vi "SW_Load_data_for_Analysis.vi"(0 "Data flow controls":T4, 1 "Cluster of paths input":T3, 4 "Progress bar reference":refnum<vi>, 5 "error in (no error)":errorcluster) -> (6 "Data column names":string[](array[string]), 7 "Stimulus presets array (loaded)":T2(array[cluster]), 8 "TTL inputs":u8[](array[numeric]), 9 "TTL outputs":u8[](array[numeric]), 10 "Absolute timestamp":dbl[](array[numeric]), 11 "Zones preference array (loaded)":dbl[][](array[numeric]), 12 "Relative timestamp":dbl[](array[numeric]), 14 "X coord":dbl[](array[numeric]), 15 "Y coord":dbl[](array[numeric]), 16 "Loaded data":T1={"Zones preference array (loaded)"=[], "TTL inputs"=[], "TTL outputs"=[], "Stimulus presets array (loaded)"=[], "Absolute timestamp"=[], "Relative timestamp"=[], "X coord"=[], "Y coord"=[], "alpha rot. angle"=[], "Current zone"=[], "Acquisition settings cluster out"={"Researcher name"="", "N segments MIDFIELD"=0, "N segments BORDER"=0, "Radius, mm CENTER"=0, "Radius, mm MIDFIELD"=0, "Starting angle MIDFIELD"=0, "Starting angle BORDER"=0, "Cage diameter, mm"=0, "Bridge swap"=FALSE, "Bridge V. offset"=0.0, "Twisted neck"=FALSE, "Offset H."=0.0, "Name prefix"="SavedTrack", "Stop at"=0.0, "\"Stop at\" enabled"=FALSE, "Settings loaded OK"=FALSE}, "Data column names"=[]} {"Acquisition settings cluster out"."Stop at" format="%<%H:%M:%S>t"}, 17 "alpha rot. angle":dbl[](array[numeric]), 18 "Current zone":dbl[](array[numeric]), 19 "error out":errorcluster)   [LabVIEW 2018, in "Tracker.lvlib"]
uses:
  <extravilib>/ChannelInstances/Stream-a[.,.](dbl)/Read With Abort.vi
  <extravilib>/ChannelInstances/Stream-a[.,.](dbl)/Write With Abort.vi
  <extravilib>/ChannelInstances/Stream-a[.,.](dbl)/EndpointRead.vi
  <extravilib>/ChannelInstances/Stream-a[.,.](dbl)/Endpoint.vi
  <vilib>/Utility/file.llb/Read Delimited Spreadsheet (string).vi
  <extravilib>/ChannelInstances/Stream-a[.,.](dbl)/Instantiate.vi
  <extravilib>/ChannelInstances/Stream-a[.,.](dbl)/)Channel.vi
  <resource>/ChannelSupport/_ChannelSupport/WaitIfNeeded.vi
  Tracker.lvlib
  <vilib>/Utility/config.llb/NI_LVConfig.lvlib
  <extravilib>/ChannelInstances/Stream-a[.,.](dbl).lvlib
panel:
  out "Settings loaded OK":bool
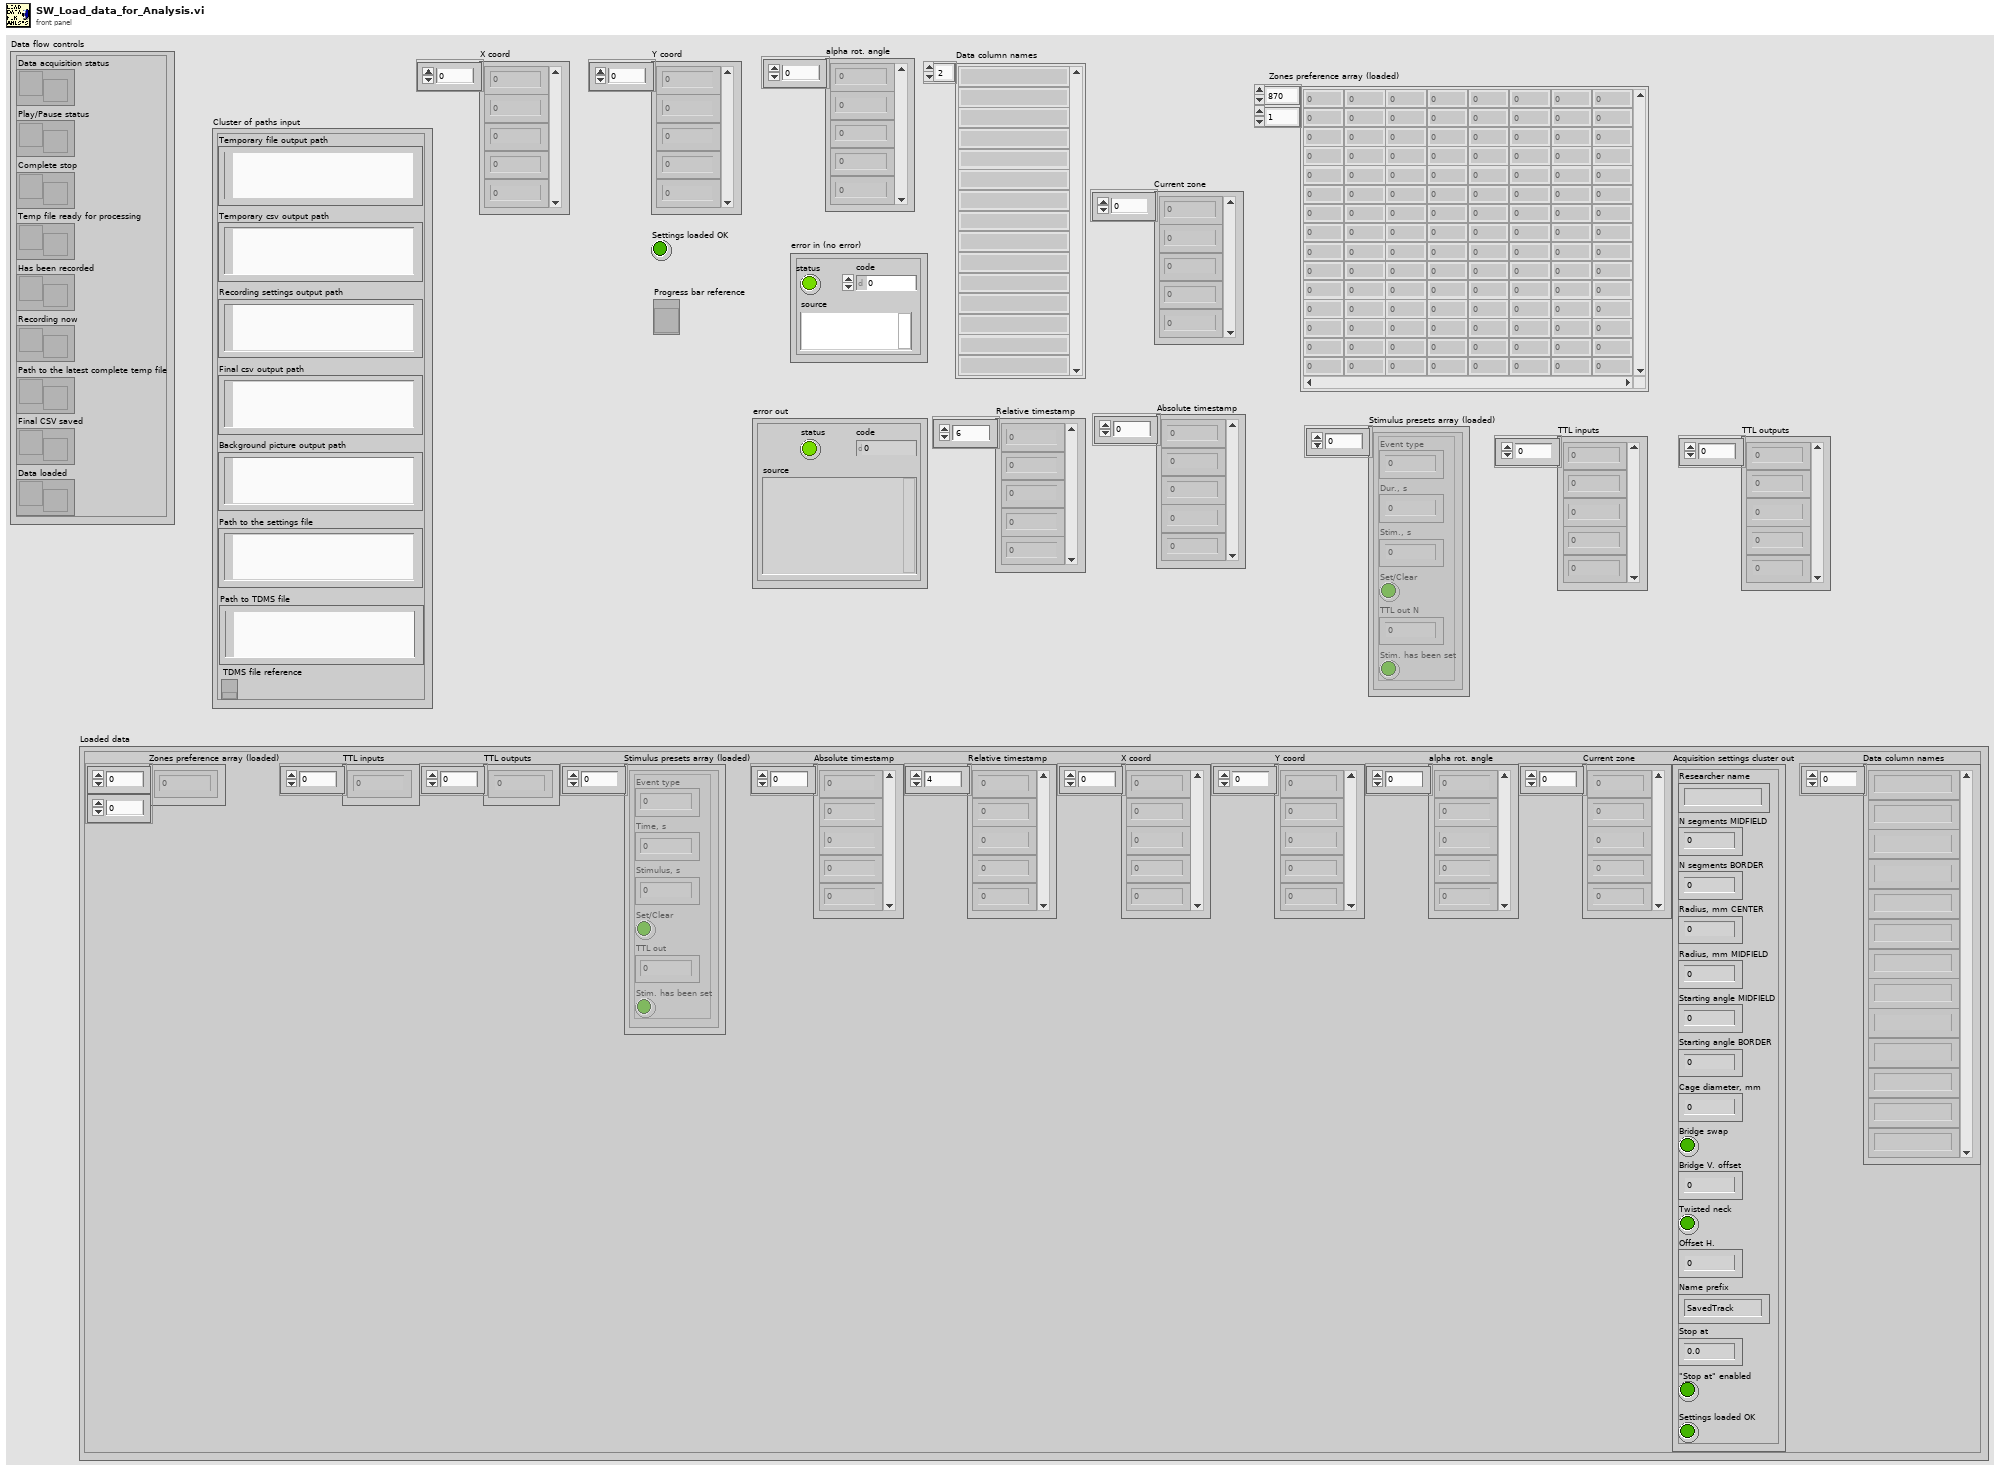
[diagram p1: front panel]
types:
  T1 = cluster{"Zones preference array (loaded)":dbl[][], "TTL inputs":u8[], "TTL outputs":u8[], "Stimulus presets array (loaded)":cluster{"Event type":u16, "Time, s":sgl, "Stimulus, s":sgl, "Set/Clear":bool, "TTL out":u16, "Stim. has been set":bool}[], "Absolute timestamp":dbl[], "Relative timestamp":dbl[], "X coord":dbl[], "Y coord":dbl[], "alpha rot. angle":dbl[], "Current zone":dbl[], "Acquisition settings cluster out":cluster{"Researcher name":string, "N segments MIDFIELD":u8, "N segments BORDER":u8, "Radius, mm CENTER":u16, "Radius, mm MIDFIELD":u16, "Starting angle MIDFIELD":i16, "Starting angle BORDER":i16, "Cage diameter, mm":u16, "Bridge swap":bool, "Bridge V. offset":sgl, "Twisted neck":bool, "Offset H.":sgl, "Name prefix":string, "Stop at":dbl, "\"Stop at\" enabled":bool, "Settings loaded OK":bool}, "Data column names":string[]}
  T2 = cluster{"Event type":u16, "Dur., s":sgl, "Stim., s":sgl, "Set/Clear":bool, "TTL out N":u16, "Stim. has been set":bool}[]
  T3 = cluster{"Temporary file output path":path, "Temporary csv output path":path, "Recording settings output path":path, "Final csv output path":path, "Background picture output path":path, "Path to the settings file":path, "Path to TDMS file":path, "TDMS file reference":refnum<k34>}
  T4 = cluster{"Data acquisition status":refnum<notifier>, "Play/Pause status":refnum<notifier>, "Complete stop":refnum<notifier>, "Temp file ready for processing":refnum<notifier>, "Has been recorded":refnum<notifier>, "Recording now":refnum<notifier>, "Path to the latest complete temp file":refnum<notifier>, "Final CSV saved":refnum<notifier>, "Data loaded":refnum<notifier>}
  T5 = typedef "NI_LVConfig.lvlib/Config Data RefNum.ctl" = refnum<k1>
  T6 = typedef "Stream-a[.,.](dbl).lvlib/)Channel.ctl" = refnum<queue>
  T7 = cluster{"Event type":u16, "Time, s":sgl, "Stimulus, s":sgl, "Set/Clear":bool, "TTL out":u16, "Stim. has been set":bool}
  T8 = cluster{"value":string, "value":u32, "value":u32, "value":u32, "value":u32, "value":i32, "value":i32, "value":u32, "value":bool, "value":dbl, bool, dbl, "key":string, dbl, bool, bool}
  T9 = cluster{"element":dbl[][], u8[], u8[], cluster{"Event type":u16, "Time, s":sgl, "Stimulus, s":sgl, "Set/Clear":bool, "TTL out":u16, "Stim. has been set":bool}[], dbl[], dbl[], dbl[], dbl[], dbl[], dbl[], cluster{"value":string, "value":u32, "value":u32, "value":u32, "value":u32, "value":i32, "value":i32, "value":u32, "value":bool, "value":dbl, bool, dbl, "key":string, dbl, bool, bool}, "first row":string[]}
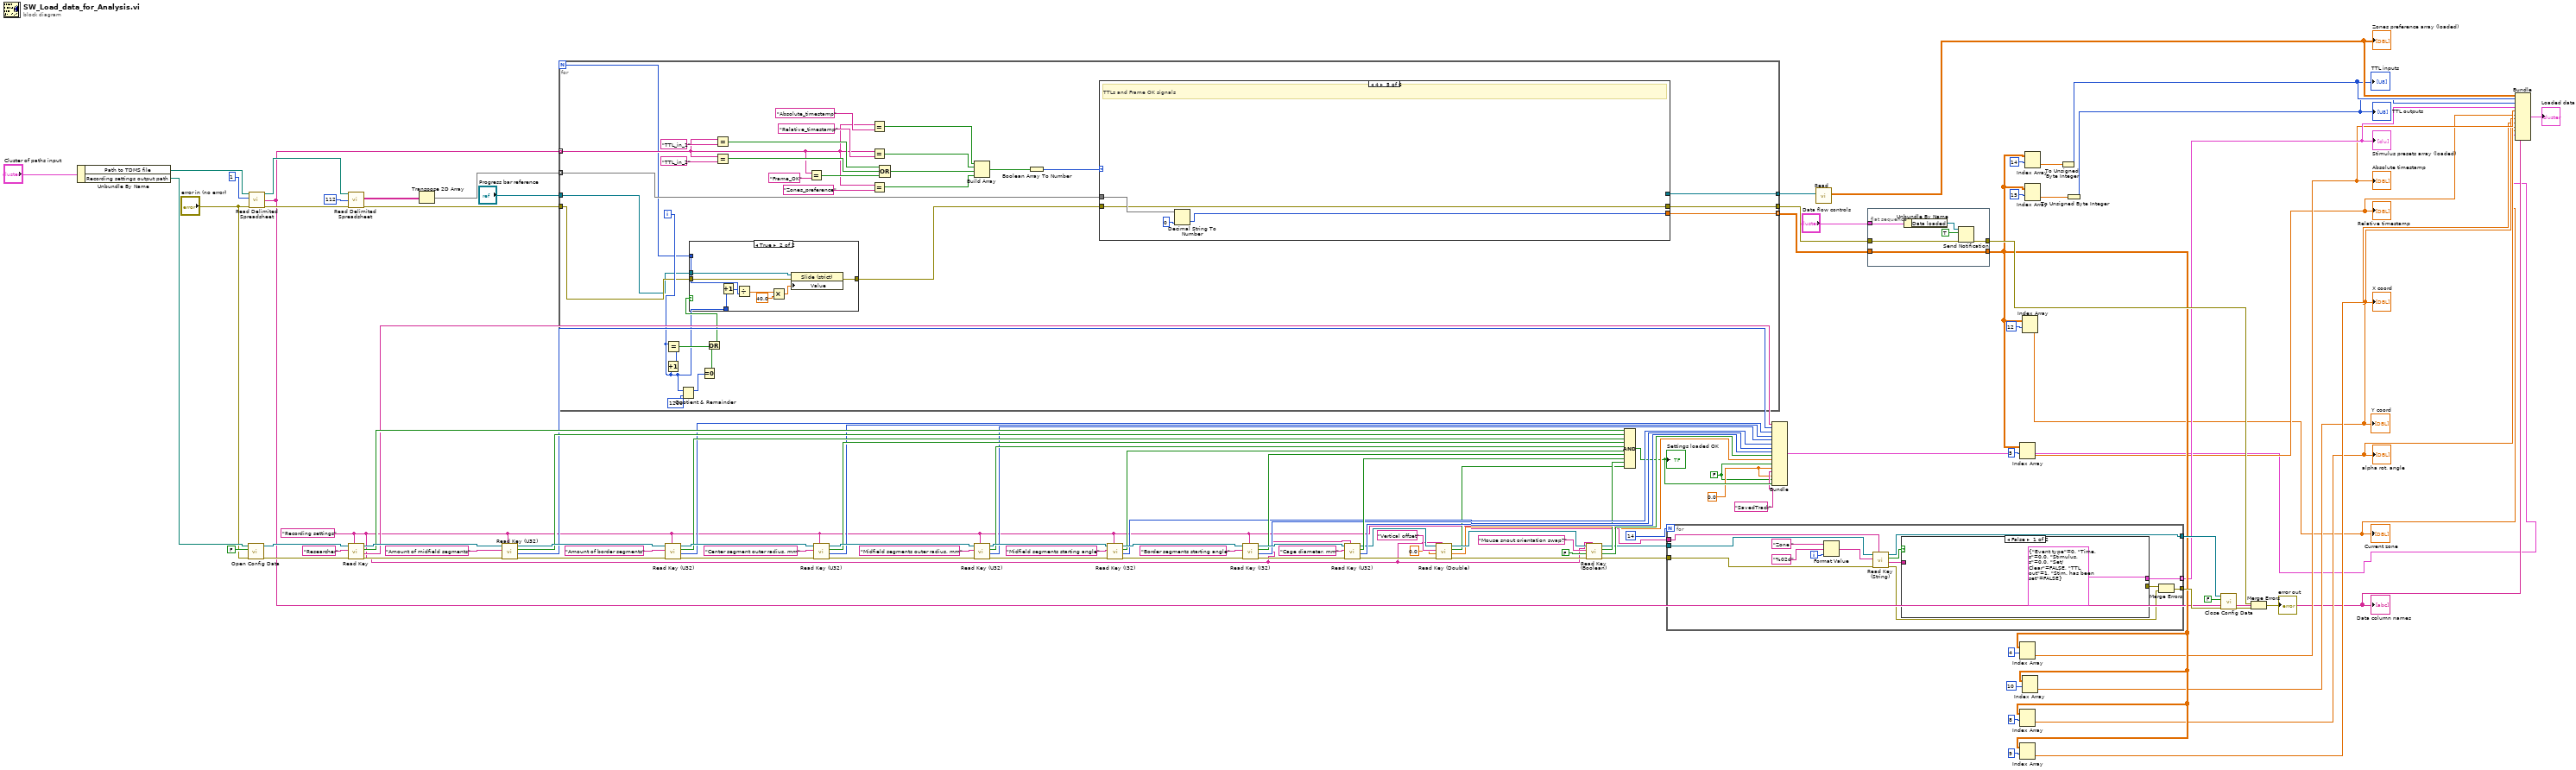
[diagram p0: block diagram]
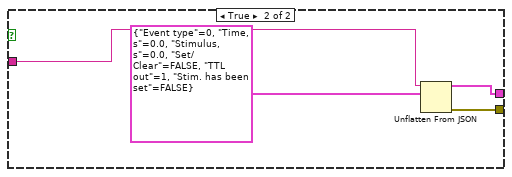
[diagram p2: hidden frame]
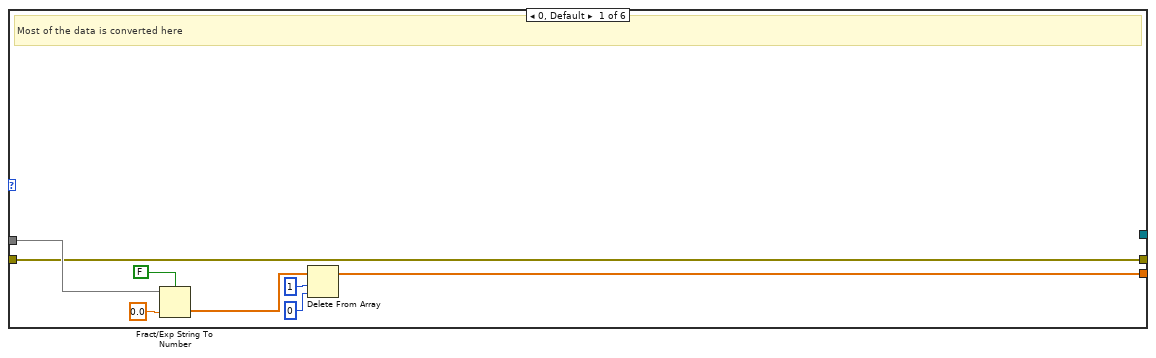
[diagram p4: hidden frame]
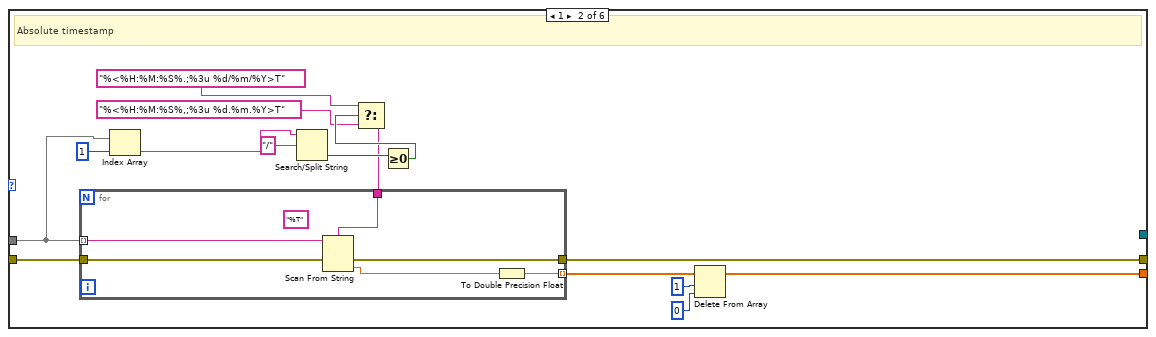
[diagram p5: hidden frame]
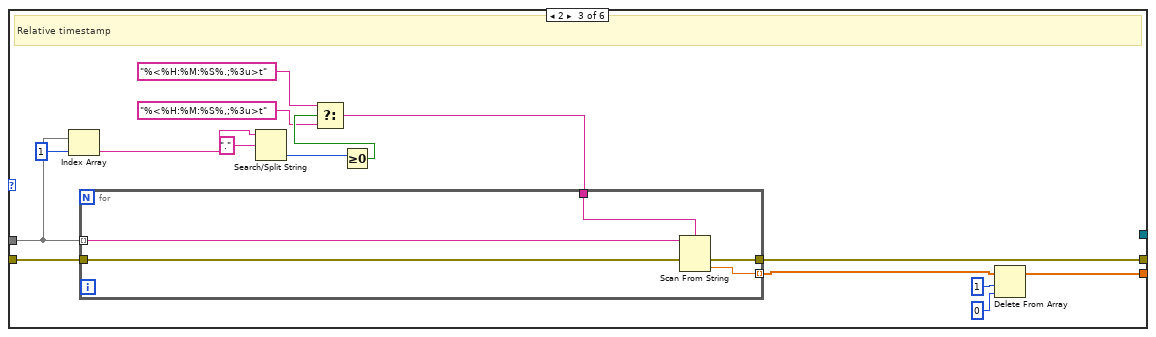
[diagram p6: hidden frame]
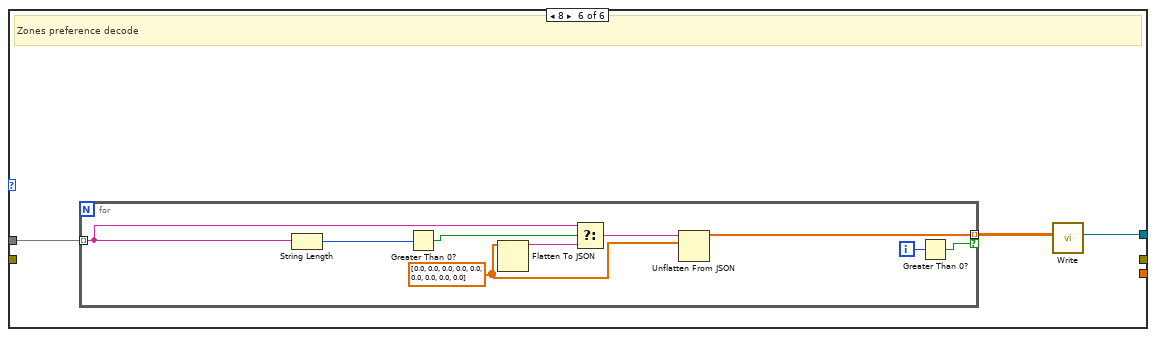
[diagram p8: hidden frame]
diagram:
  w3 = 0.0
  w2 = FALSE
  w25 = "Recording settings" ("section")
  n1 = Unbundle By Name("Cluster of paths input") -> ("Path to TDMS file"=w100:path, "Recording settings output path"=w91:path)
  n2 = call <vilib>:"Open Config Data.vi"("error in (no error)"="error in (no error)", "create file if necessary (T)"=FALSE, "configuration file path"=w91) -> ("error out"=w66:errorcluster, "refnum"=w89:T5)  [unwired: 6 in, 1 out]
  n3 = call-poly <vilib>:"Read Delimited Spreadsheet.vi"("file path (dialog if empty)"=w100, "number of rows (all:-1)"=1, "error in (no error)"="error in (no error)") -> ("new file path (Not A Path if cancelled)"=w102:path, "first row"=w7:string[], "error out"=w105:errorcluster)  [unwired: 7 in, 3 out]
  "Data column names" <- w7
  n4 = call-poly <vilib>:"Read Delimited Spreadsheet.vi"("file path (dialog if empty)"=w102, "start of read offset (chars.:0)"=112, "error in (no error)"=w105) -> ("all rows"=w103:string[][], "error out"=w96:errorcluster)  [unwired: 7 in, 4 out]
  n5 = call-poly <vilib>:"Read Key.vi"("section"=w25, "error in (no error)"=w66, "key"="Researcher", "refnum"=w89) -> ("error out"=w85:errorcluster, "value"=w52:string, "found?"=w65:bool, "refnum out"=w87:T5)  [unwired: 4 in]
  n6 = Transpose 2D Array(2D array=w103) -> (transposed array=w101:string[][])
  n7 = call <vilib>:"Read Key (U32).vi"("section"=w25, "error in (no error)"=w85, "key"="Amount of midfield segments", "refnum"=w87) -> ("error out"=w83:errorcluster, "value"=w51:u32, "found?"=w64:bool, "refnum out"=w84:T5)  [unwired: 4 in]
  n8 = for {
    N -> [w108]
    tunnel: w7 -> [w122] mode=indexing
    tunnel: w101 -> [w119] mode=indexing
    tunnel: [w125] -> w94 mode=indexing
    tunnel: w96 -> [w110]
    tunnel: [w124] -> w95
    tunnel: "Progress bar reference" -> [w109]
    tunnel: [w120] -> w37
    i -> [w111]
    n9 = Increment(x=w111) -> (x+1=w118:i32)
    n10 = Equal?(x=w111, y=w118) -> (x = y?=w117:bool)
    n11 = Quotient & Remainder(x=w111, y=1200) -> (x-y*floor(x/y)=w114:i32)  [unwired: 1 out]
    n12 = Equal To 0?(x=w114) -> (x = 0?=w115:bool)
    n13 = Or(x=w117, y=w115) -> (x .or. y?=w116:bool)
    n14 = case shown="True" w116 {
      tunnel: w111 -> [_ w148]
      tunnel: w108 -> [_ w147]
      tunnel: w109 -> [_ w146]
      tunnel: w110 -> [w139 w145]
      tunnel: [w139 w144] -> w112
      frame False {
      }
      frame True {
        n15 = Increment(x=w148) -> (x+1=w141:i32)
        n16 = Divide(x=w141, y=w147) -> (x/y=w143:dbl)
        n17 = Multiply(x=w143, y=40.0) -> (x*y=w140:dbl)
        n18 = property on="Property Node" class="Slide (strict)"(reference=w146, error in=w145, "Value"=w140) -> (error out=w144:errorcluster)  [unwired: 1 out]
      }
    }
    n19 = Equal?(x=w122, y="TTL_in_1") -> (x = y?=w133:bool)
    n20 = Equal?(x=w122, y="TTL_in_2") -> (x = y?=w132:bool)
    n21 = Equal?(x=w122, y="Frame_OK") -> (x = y?=w131:bool)
    n22 = Equal?(x=w122, y="Absolute_timestamp") -> (x = y?=w126:bool)
    n23 = Equal?(x=w122, y="Relative_timestamp") -> (x = y?=w127:bool)
    n24 = Equal?(x=w122, y="Zones_preference") -> (x = y?=w121:bool)
    n25 = Compound Arithmetic op=OR(w133, w132, w131) -> (w130:bool)
    n26 = Build Array(w126, w127, w130, w121) -> (w129:bool[])
    n27 = Boolean Array To Number(Boolean array=w129) -> (number=w128:u32)
    n28 = case shown="4" w128 {
      tunnel: w119 -> [w156 w160 w186 _ w202 w205]
      tunnel: [w149 w166 w187 _ w200 _] -> w125
      tunnel: w112 -> [w153 w171 w192 w198 w199 _]
      tunnel: [w153 w170 w191 w198 w199 _] -> w124
      tunnel: [_ _ _ _ _ w203] -> w120
      frame 0, Default {
        # "Most of the data is converted here"
        n29 = Fract/Exp String To Number(use system decimal point (T)=FALSE, string=w156, default (0 dbl)=0.0 ("default (0 DBL)")) -> (number=w152:dbl[])  [unwired: 1 in, 1 out]
        n30 = Delete From Array(array=w152, length=1, index=0) -> (array with subset deleted=w149:dbl[])  [unwired: 1 out]
      }
      frame 1 {
        # "Absolute timestamp"
        n31 = Index Array(array=w160, index=1) -> (element=w161:string)
        n32 = Search/Split String(string=w161, search string/char (-)="/") -> (offset of match=w163:i32)  [unwired: 1 in, 2 out]
        n33 = Greater Or Equal To 0?(x=w163) -> (x >= 0?=w164:bool)
        n34 = Select(t="%<%H:%M:%S%.;%3u %d/%m/%Y>T" ("format string"), s=w164, f="%<%H:%M:%S%,;%3u %d.%m.%Y>T" ("format string")) -> (s? t:f=w159:string)
        n35 = for {
          tunnel: w160 -> [w177] mode=indexing
          tunnel: [w175] -> w167 mode=indexing
          tunnel: w171 -> [w174]
          tunnel: [w173] -> w170
          tunnel: w159 -> [w172]
          (unwired) "%T" ("format string")
          n36 = Scan From String(format string=w172, input string=w177, error in=w174) -> (error out=w173:errorcluster, output 1=w176:dbl)  [unwired: 2 in, 2 out]
          n37 = To Double Precision Float(number=w176) -> (double precision float=w175:dbl)
        }
        n38 = Delete From Array(array=w167, length=1, index=0) -> (array with subset deleted=w166:dbl[])  [unwired: 1 out]
      }
      frame 2 {
        # "Relative timestamp"
        n39 = Index Array(array=w186, index=1) -> (element=w179:string)
        n40 = Search/Split String(string=w179, search string/char (-)=".") -> (offset of match=w181:i32)  [unwired: 1 in, 2 out]
        n41 = Greater Or Equal To 0?(x=w181) -> (x >= 0?=w184:bool)
        n42 = Select(t="%<%H:%M:%S%.;%3u>t" ("format string"), s=w184, f="%<%H:%M:%S%,;%3u>t" ("format string")) -> (s? t:f=w178:string)
        n43 = for {
          tunnel: w186 -> [w197] mode=indexing
          tunnel: [w196] -> w188 mode=indexing
          tunnel: w192 -> [w195]
          tunnel: [w194] -> w191
          tunnel: w178 -> [w193]
          n44 = Scan From String(format string=w193, input string=w197, error in=w195) -> (error out=w194:errorcluster, output 1=w196:dbl)  [unwired: 2 in, 2 out]
        }
        n45 = Delete From Array(array=w188, length=1, index=0) -> (array with subset deleted=w187:dbl[])  [unwired: 1 out]
      }
      frame 3 {
      }
      frame 4 {
        # "TTLs and Frame OK signals"
        n46 = Decimal String To Number(string=w202, default (0L)=u8 0 ("default (0 I32)")) -> (number=w200:u8[])  [unwired: 1 in, 1 out]
      }
      frame 8 {
        # "Zones preference decode"
        n47 = for {
          tunnel: w205 -> [w211] mode=indexing
          tunnel: [w208] -> w204 mode=indexing if=w207
          i -> [w206]
          w209 = dbl[] [0.0, 0.0, 0.0, 0.0, 0.0, 0.0, 0.0, 0.0, 0.0] ("Zones normalized allocation array")
          n48 = String Length(string=w211) -> (length=w214:i32)
          n49 = Greater Than 0?(x=w214) -> (x > 0?=w213:bool)
          n50 = Flatten To JSON(anything=w209) -> (JSON string=w210:string)  [unwired: 2 in, 1 out]
          n51 = Select(t=w211, s=w213, f=w210) -> (s? t:f=w212:string)
          n52 = Unflatten From JSON(JSON string=w212, type and defaults=w209) -> (value=w208:dbl[])  [unwired: 5 in, 1 out]
          n53 = Greater Than 0?(x=w206) -> (x > 0?=w207:bool)
        }
        n54 = call <extravilib>:"Write.vi"("element"=w204) -> ("channel"=w203:T6)  [unwired: 8 in, 2 out]
      }
    }
  }
  n55 = call <vilib>:"Read Key (U32).vi"("section"=w25, "error in (no error)"=w83, "key"="Amount of border segments", "refnum"=w84) -> ("error out"=w81:errorcluster, "value"=w50:u32, "found?"=w63:bool, "refnum out"=w74:T5)  [unwired: 4 in]
  n56 = call <vilib>:"Read Key (U32).vi"("section"=w25, "error in (no error)"=w81, "key"="Center segment outer radius, mm", "refnum"=w74) -> ("error out"=w80:errorcluster, "value"=w49:u32, "found?"=w62:bool, "refnum out"=w73:T5)  [unwired: 4 in]
  n57 = call <vilib>:"Read Key (U32).vi"("section"=w25, "error in (no error)"=w80, "key"="Midfield segments outer radius, mm", "refnum"=w73) -> ("error out"=w79:errorcluster, "value"=w48:u32, "found?"=w61:bool, "refnum out"=w72:T5)  [unwired: 4 in]
  n58 = call <vilib>:"Read Key (I32).vi"("section"=w25, "error in (no error)"=w79, "key"="Midfield segments starting angle", "refnum"=w72) -> ("error out"=w78:errorcluster, "value"=w47:i32, "found?"=w60:bool, "refnum out"=w71:T5)  [unwired: 4 in]
  n59 = call <vilib>:"Read Key (I32).vi"("section"=w25, "error in (no error)"=w78, "key"="Border segments starting angle", "refnum"=w71) -> ("error out"=w77:errorcluster, "value"=w46:i32, "found?"=w59:bool, "refnum out"=w70:T5)  [unwired: 4 in]
  n60 = call <vilib>:"Read Key (U32).vi"("section"=w25, "error in (no error)"=w77, "key"="Cage diameter, mm", "refnum"=w70) -> ("error out"=w36:errorcluster, "value"=w45:u32, "found?"=w58:bool, "refnum out"=w34:T5)  [unwired: 4 in]
  n61 = call <vilib>:"Read Key (Double).vi"("section"=w25, "error in (no error)"=w36, "default value"=0.0, "key"="Vertical offset", "refnum"=w34) -> ("error out"=w35:errorcluster, "value"=w29:dbl, "found?"=w30:bool, "refnum out"=w33:T5)  [unwired: 3 in]
  n62 = call <vilib>:"Read Key (Boolean).vi"("section"=w25, "error in (no error)"=w35, "default value"=FALSE, "key"="Mouse snout orientation swap?", "refnum"=w33) -> ("error out"=w27:errorcluster, "value"=w40:bool, "found?"=w41:bool, "refnum out"=w24:T5)  [unwired: 3 in]
  n63 = Compound Arithmetic op=AND(w65, w64, w63, w62, w61, w60, w59, w58, w41, w30) -> (w5:bool)
  "Settings loaded OK" <- w5
  n64 = for {
    N: 14 -> [_]
    tunnel: w24 -> [w226]
    tunnel: [w225] -> w23
    tunnel: w25 -> [w224]
    tunnel: w27 -> [w222]
    tunnel: [w216] -> w26
    tunnel: [w219] -> w14 mode=indexing
    i -> [w217]
    n65 = Format Value(string ("")="Zone ", format string="%02d", value (0)=w217) -> (output string=w223:string)
    n66 = call <vilib>:"Read Key (String).vi"("section"=w224, "error in (no error)"=w222, "key"=w223, "refnum"=w226) -> ("error out"=w221:errorcluster, "value"=w220:string, "found?"=w218:bool, "refnum out"=w225:T5)  [unwired: 4 in]
    n67 = case shown="False" w218 {
      tunnel: w220 -> [_ w233]
      tunnel: [T7 {"Event type"=0, "Time, s"=0.0, "Stimulus, s"=0.0, "Set/Clear"=FALSE, "TTL out"=1, "Stim. has been set"=FALSE} ("Cluster of the stimuls settings") w232] -> w219
      tunnel: [_ w231] -> w215
      frame False {
      }
      frame True {
        n68 = Unflatten From JSON(JSON string=w233, type and defaults=T7 {"Event type"=0, "Time, s"=0.0, "Stimulus, s"=0.0, "Set/Clear"=FALSE, "TTL out"=1, "Stim. has been set"=FALSE} ("Cluster of the stimuls settings")) -> (value=w232:T7, error out=w231:errorcluster)  [unwired: 5 in]
      }
    }
    n69 = Merge Errors(w215, w221) -> (w216:errorcluster)
  }
  "Stimulus presets array (loaded)" <- w14
  n70 = Bundle("value"=w52, "value"=w51, "value"=w50, "value"=w49, "value"=w48, "value"=w47, "value"=w46, "value"=w45, "value"=w40, "value"=w29, w2, w3, "key"="SavedTrack", w3, w2, w5) -> (w1:T8)  [unwired: 1 in]
  n71 = call <extravilib>:"Read.vi"("channel"=w37) -> ("element"=w17:dbl[][])  [unwired: 6 in, 4 out]
  "Zones preference array (loaded)" <- w17
  n72 = flat-sequence {
    tunnel: w94 -> [w239]
    tunnel: [w239] -> w18
    tunnel: "Data flow controls" -> [w236]
    tunnel: [w235] -> w76
    tunnel: w95 -> [w234]
    frame #0 {
      n73 = Unbundle By Name(w236) -> ("Data loaded"=w237:refnum<notifier>)
      n74 = Send Notification(notification=TRUE, notifier=w237, error in (no error)=w234) -> (error out=w235:errorcluster)  [unwired: 1 out]
    }
  }
  n75 = Index Array(array=w18, index (row)=5 ("disabled index (col)")) -> (element=w12:dbl[])  [unwired: 1 in]
  "Relative timestamp" <- w12
  n76 = Index Array(array=w18, index (row)=4 ("disabled index (col)")) -> (element=w13:dbl[])  [unwired: 1 in]
  "Absolute timestamp" <- w13
  n77 = Index Array(array=w18, index (row)=8) -> (element=w9:dbl[])  [unwired: 1 in]
  "alpha rot. angle" <- w9
  n78 = Index Array(array=w18, index (row)=9 ("disabled index (col)")) -> (element=w11:dbl[])  [unwired: 1 in]
  "X coord" <- w11
  n79 = Index Array(array=w18, index (row)=12) -> (element=w8:dbl[])  [unwired: 1 in]
  "Current zone" <- w8
  n80 = Index Array(array=w18, index (row)=10) -> (element=w10:dbl[])  [unwired: 1 in]
  "Y coord" <- w10
  n81 = Index Array(array=w18, index (row)=14) -> (element=w22:dbl[])  [unwired: 1 in]
  n82 = Index Array(array=w18, index (row)=15) -> (element=w19:dbl[])  [unwired: 1 in]
  n83 = To Unsigned Byte Integer(number=w22) -> (unsigned 8bit integer=w16:u8[])
  "TTL inputs" <- w16
  n84 = To Unsigned Byte Integer(number=w19) -> (unsigned 8bit integer=w15:u8[])
  "TTL outputs" <- w15
  n85 = call <vilib>:"Close Config Data.vi"("error in (no error)"=w26, "write file if changed (T)"=FALSE, "refnum"=w23) -> ("error out"=w69:errorcluster)  [unwired: 7 in, 1 out]
  n86 = Merge Errors(w76, w69) -> (→"error out":errorcluster)
  n87 = Bundle("element"=w17, w16, w15, w14, w13, w12, w11, w10, w9, w8, w1, "first row"=w7) -> (→"Loaded data":T9)  [unwired: 1 in]
